vi "SVD.vi"() -> ()   [LabVIEW 2017]
uses:
  <vilib>/Analysis/Matrix/Datatypes/RealMatrix.ctl
  <vilib>/Analysis/7linalg.llb/SVD Option.ctl
  <vilib>/Analysis/7linalg.llb/Real Transpose Matrix.vi
  <vilib>/Analysis/7linalg.llb/Real SVD Decomposition.vi
  <vilib>/Analysis/NI_AALPro.lvlib
  <vilib>/Analysis/Matrix/NI_Matrix.lvlib
panel:
  out "Saving Data":bool
  in  "?":bool
  out "V Transpose":T1
  out "Matrix V":T1
  out "Matrix S":T1
  out "Matrix U":T1
  out "Vector S":dbl[](array[numeric])
  in  "SVD option":T2 items=["Thin", "Full"]
  in  "singular values only?":bool
  in  "A":T1
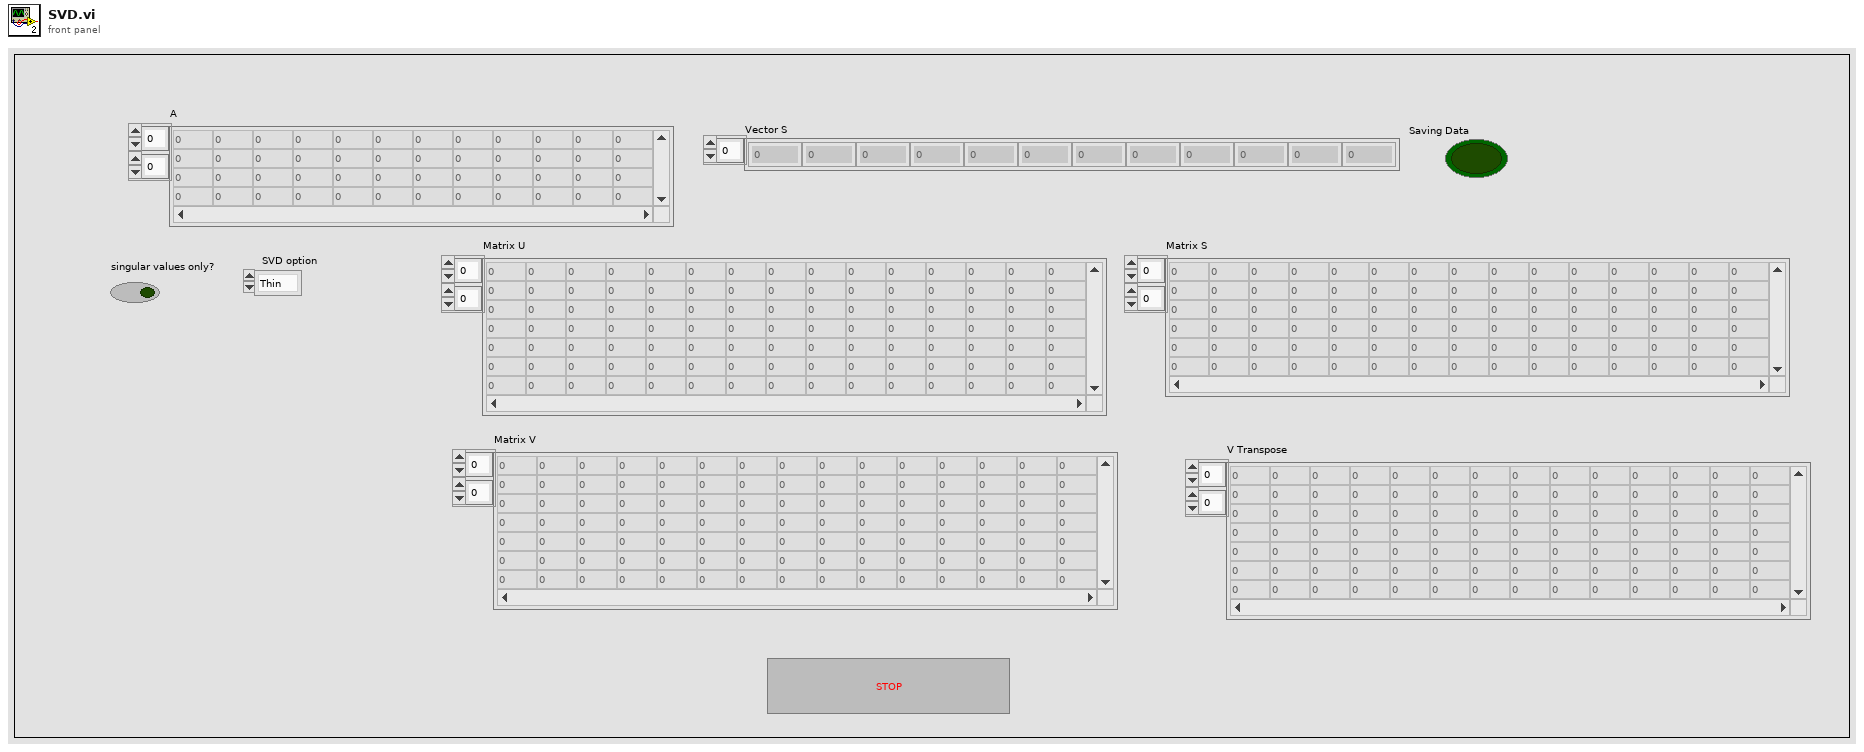
[diagram p1: front panel]
types:
  T1 = typedef "NI_Matrix.lvlib/RealMatrix.ctl" = dbl[][]
  T2 = typedef "NI_AALPro.lvlib/SVD Option.ctl" = u16
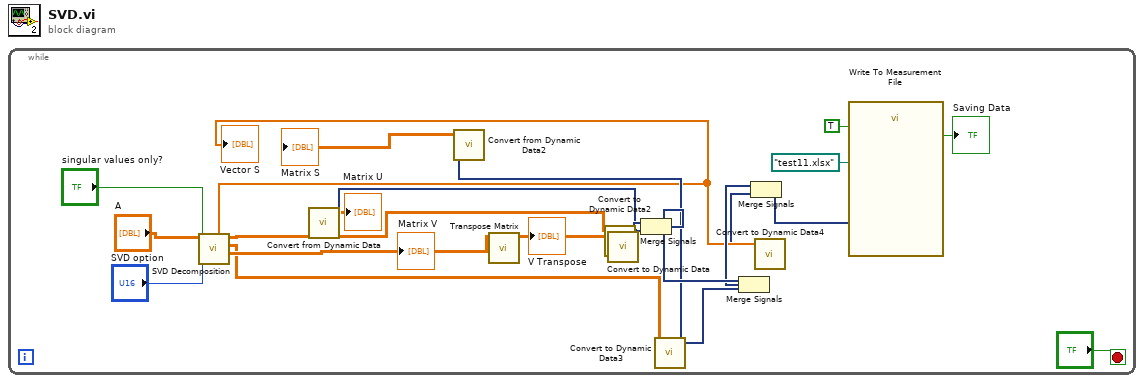
[diagram p0: block diagram]
diagram:
  n1 = while {
    stop <- "?" stop-if-true
    n2 = call-poly <vilib>:"SVD Decomposition.vi"("SVD option"="SVD option", "singular values only?"="singular values only?", "A"="A") -> ("Matrix V"=w18:T1, "Matrix S"=w10:T1, "Matrix U"=w14:T1, "Vector S"=w6:dbl[])  [unwired: 4 in, 1 out]
    "Vector S" <- w6
    "Matrix V" <- w18
    n3 = call-poly <vilib>:"Transpose Matrix.vi"("Input Matrix"=w18) -> ("Matrix Transpose"=w17:T1)  [unwired: 9 in, 1 out]
    "V Transpose" <- w17
    n4 = call "Convert to Dynamic Data2"("2D Array"=w14) -> ("Dynamic Data Type"=w13:dynamicdata)  [unwired: 3 in]
    n5 = call "Convert from Dynamic Data"("Dynamic Data Type"=w13) -> ("Array"=→"Matrix U":dbl[][])  [unwired: 3 in]
    n6 = call "Convert to Dynamic Data"("2D Array"=w17) -> ("Dynamic Data Type"=w16:dynamicdata)  [unwired: 3 in]
    n7 = Merge Signals(w16, w13) -> (w15:dynamicdata)
    n8 = call "Convert to Dynamic Data3"("2D Array"=w10) -> ("Dynamic Data Type"=w9:dynamicdata)  [unwired: 3 in]
    n9 = call "Convert from Dynamic Data2"("Dynamic Data Type"=w9) -> ("Array"=→"Matrix S":dbl[][])  [unwired: 3 in]
    n10 = Merge Signals(w15, w9) -> (w11:dynamicdata)
    n11 = call "Convert to Dynamic Data4"("Array"=w6) -> ("Dynamic Data Type"=w5:dynamicdata)  [unwired: 3 in]
    n12 = Merge Signals(w11, w5) -> (w7:dynamicdata)
    n13 = call "Write To Measurement File"("Signals"=w7, "Enable"=TRUE, "Filename"=path "test11.xlsx") -> ("Saving Data"=→"Saving Data":bool)  [unwired: 14 in, 2 out]
  }
